vi "Engine UI Msg Callback.vi"(4 "User Parameter":variant, 5 "Event Data":cluster{"msg":refnum<k7>}, 6 "Control Ref":refnum<k7>, 7 "Event Common Data":T1) -> ()   [LabVIEW 2020, in "HTS.lvlib" / "Engine.lvclass"]
uses:
  Engine.lvclass
  Data Types/UIMsg.ctl
  Engine.lvclass/Engine.ctl
  HTS.lvlib
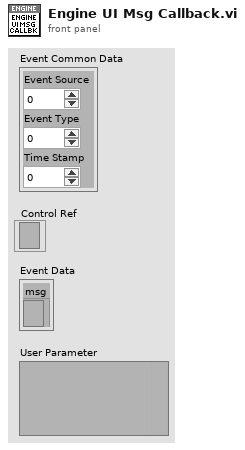
[diagram p1: front panel]
types:
  T1 = cluster{"Event Source":i32, "Event Type":u32, "Time Stamp":u32}
  T2 = typedef "HTS.lvlib/UIMsg.ctl" = enum16{"Unknown", "BreakOnUserRequest", "BreakOnBreakpoint", "BreakOnRunTimeError", "Trace", "TerminatingExecution", "AbortingExecution", "KillingExecutionThreads", "EndExecution", "ShutDownComplete", "StartExecution", "ProgressPercent", "ProgressText", "StartInteractiveExecution", "EndInteractiveExecution", "TerminatingInteractiveExecution", "TerminationCancelled", "ResumeFromBreak", "StartFileExecution", "EndFileExecution", "ShutDownCancelled", "LocalizationSettingChanged", "OpenWindows", "TileWindows", "CascadeWindows", "ReportChanged", "CloseWindows", "RefreshWindows", "ClientFileChanged", "DisplayReport", "ModelState_Initializing", "ModelState_Waiting", "ModelState_Identified", "ModelState_BeginTesting", "ModelState_TestingComplete", "ModelState_PostProcessingComplete", "ModelState_EnabledStateSet", "ReportLocationChanged", "GotoLocation", "PushUndoItem", "OutputMessages", "TypePaletteFileListChanged", "NonTerminatingThreadsArePreventingTermination", "ModelState_PostProcessing", "ReportCollectionChanged", "RuntimeError"}
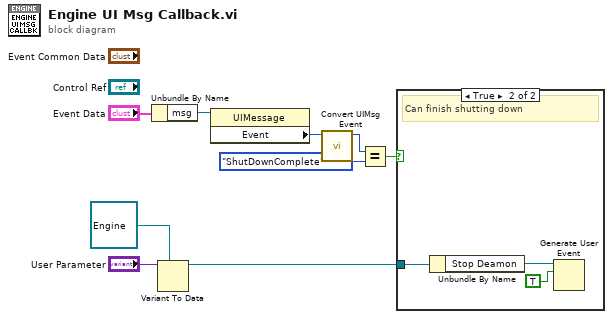
[diagram p0: block diagram]
diagram:
  n1 = Unbundle By Name("Event Data") -> ("msg"=w8:refnum<k7>)
  n2 = Variant To Data(type=refnum<class "Engine.lvclass"> refnum ("TSEngine"), Variant="User Parameter") -> (data=w4:refnum<class "Engine.lvclass">)  [unwired: 1 in, 1 out]
  n3 = property class="UIMessage"(reference=w8) -> ("Event"=w3:i32)  [unwired: 1 in, 2 out]
  n4 = call "Convert UIMsg Event.vi"("UIMsg Event"=w3) -> ("UIMsg"=w2:T2)  [unwired: 9 in, 1 out]
  n5 = Equal?(x=w2, y=UIMsg."ShutDownComplete") -> (x = y?=w5:bool)
  n6 = case shown="True" w5 {
    tunnel: w4 -> [_ w12]
    frame False {
    }
    frame True {
      # "Can finish shutting down"
      n7 = Unbundle By Name(w12) -> ("Stop Deamon"=w11:refnum<user-event>)
      n8 = Generate User Event(user event=w11, event data cluster=TRUE ("event data")) -> ()  [unwired: 2 in, 2 out]
    }
  }
